vi "TestCHampSonde(2C).vi"(0 "Range":dbl=52.8 format="%.2f", 1 "CentreTel X":i32=647041 min=0 max=1000000 step=1000, 3 "PulsexCentre":i32=641444 min=0 max=1000000 step=1000, 5 "ParametresInstrumentaux":string[](array[string]), 9 "Rot(rad)":dbl=3.6441621315637374 step=0.1 format="%.2f", 11 "acrmin/pulse":dbl=5.28e-05 format="%.4e", 12 "CentreTel Y":i32=70736 min=0 max=1000000 step=1000, 14 "PulseyCentre":i32=41801 min=0 max=1000000 step=1000) -> (4 "Champ":cluster{dbl[], dbl[]}[](array[cluster])=[{[5.0, 5.0], [5.0, -5.0]}, {[5.0, -5.0], [-5.0, -5.0]}, {[-5.0, -5.0], [-5.0, 5.0]}, {[-5.0, 5.0], [5.0, 5.0]}, {[40.96033829233336, 15.527693293631083], [-35.21795510048486, 11.053208364139456]}, {[15.527693293631083, -30.74347017099323], [11.053208364139456, -14.37943663456282]}, {[-30.74347017099323, -5.310825172290953], [-14.37943663456282, -60.65060009918713]}, {[40.96033829233336, -5.310825172290953], [-35.21795510048486, -60.65060009918713]}, {array[360 elements], array[360 elements]}] {"?" format="%.2f"; "?" format="%.2f"}, 6 "offRA":dbl=0.9948732849489528 format="%.2f", 8 "rayon de sécurité ...":dbl, 10 "offDEC":dbl=-1.196509600791168 format="%.2f")   [LabVIEW 2010]
panel:
  out "p2y":dbl
  out "p2x":dbl
  out "p1y":dbl
  out "p1x":dbl
  out "XY Graph":cluster{dbl[], dbl[]}[](graph)
  # "Exclusion y1"
  # "Exclusion y2"
  # "Champ"
  # "Exclusion x1"
  # "Exclusion x2"
  # "foyerTel"
  # "foyerSonde"
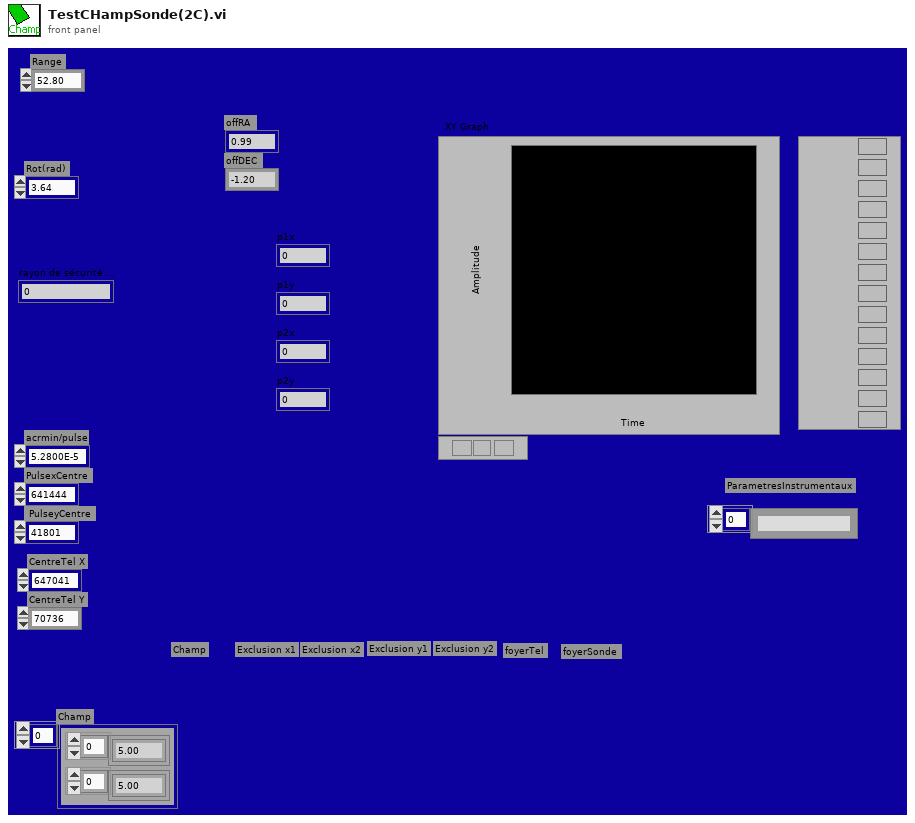
[diagram p1: front panel]
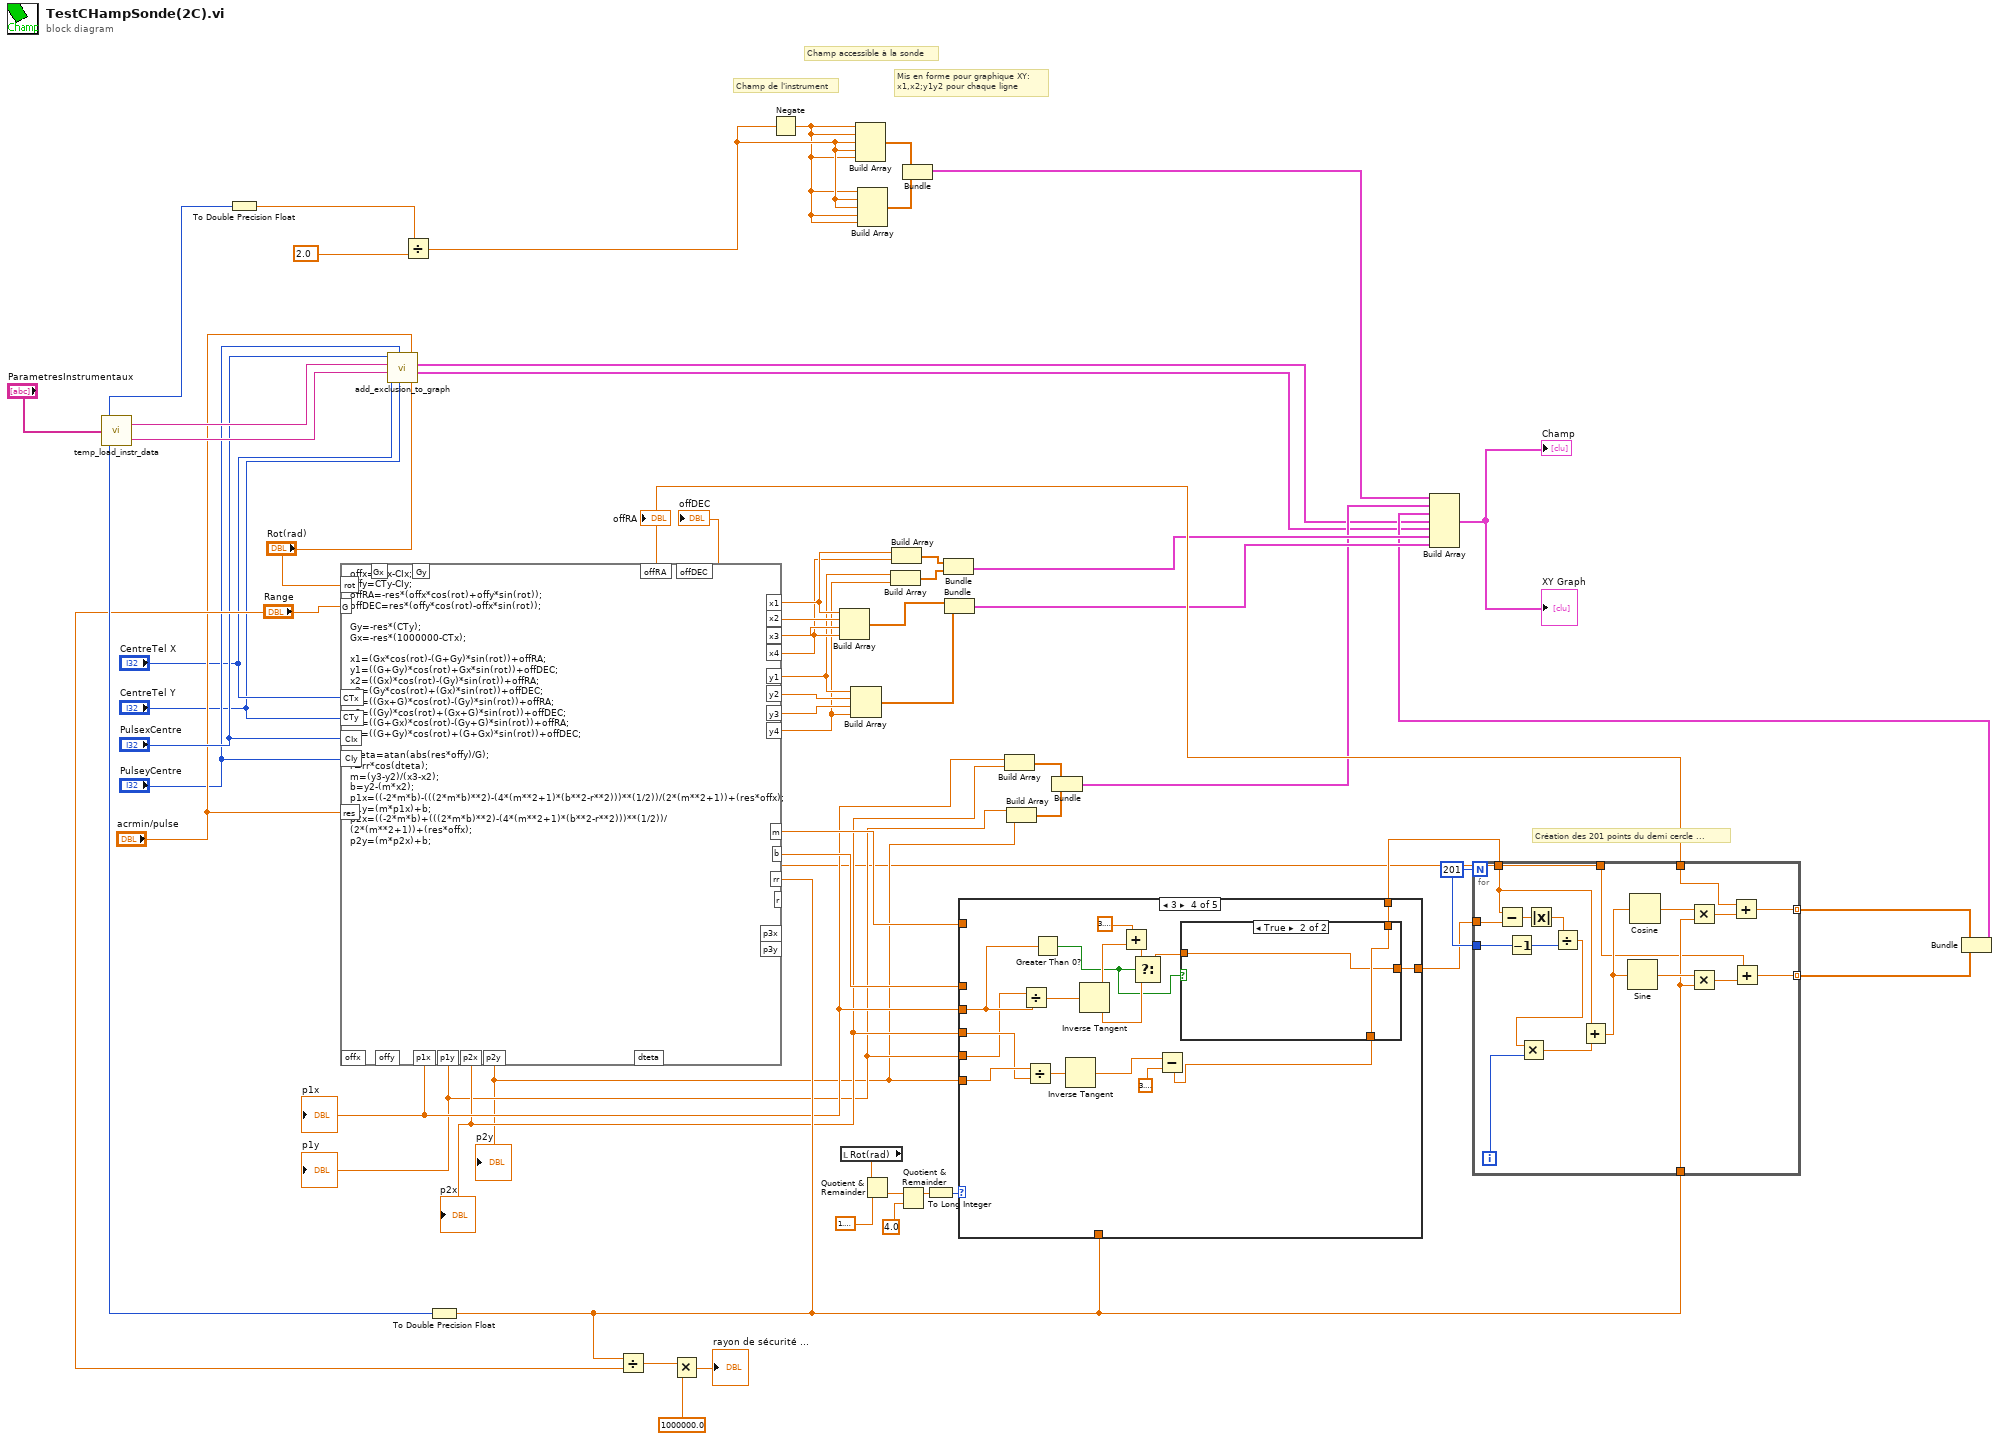
[diagram p0: block diagram]
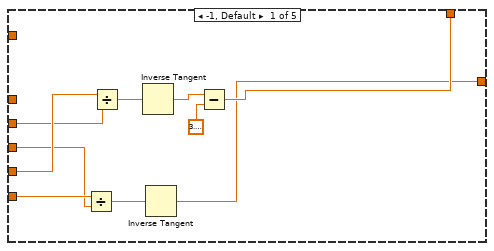
[diagram p2: hidden frame]
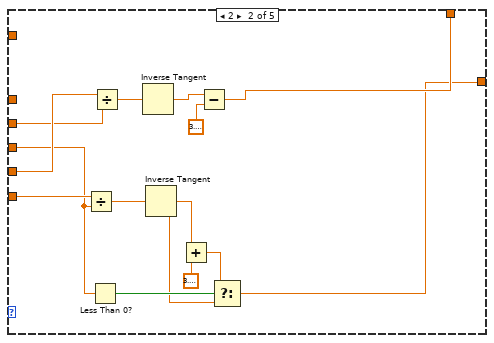
[diagram p3: hidden frame]
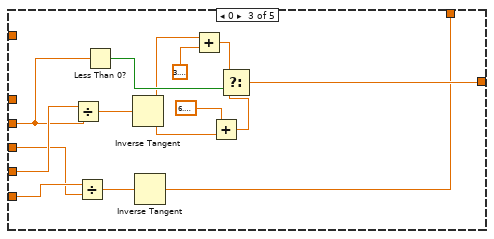
[diagram p4: hidden frame]
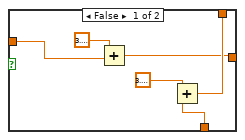
[diagram p5: hidden frame]
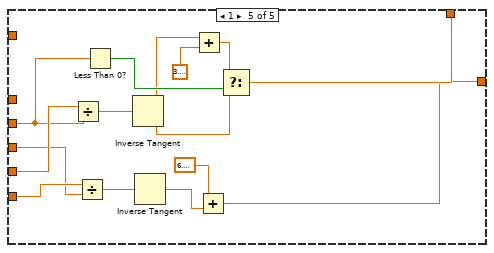
[diagram p6: hidden frame]
diagram:
  w59 = 201
  # "Création des 201 points du demi cercle ..."
  # "Champ accessible à la sonde"
  # "Champ de l'instrument"
  # "Mis en forme pour graphique XY:\nx1,x2;y1y2 pour chaque ligne"
  n1 = call "temp_load_instr_data.vi"("ParametresInstrumentaux"="ParametresInstrumentaux") -> ("2e couple"=w10:string, "1er couple"=w9:string, "rayon"=w46:i32, "champ"=w48:i32)
  n2 = To Double Precision Float(number=w48) -> (double precision float=w47:dbl)
  n3 = call "add_exclusion_to_graph.vi"("Rot(rad)"="Rot(rad)", "acrmin/pulse"="acrmin/pulse", "CentreTel Y"="CentreTel Y", "PulseyCentre"="PulseyCentre", "CentreTel X"="CentreTel X", "2er couple"=w10, "1er couple"=w9, "PulsexCentre"="PulsexCentre") -> ("Cavenas"=w1:cluster{dbl[], dbl[]}, "line one"=w2:cluster{dbl[], dbl[]})
  n4 = Divide(x=w47, y=2.0) -> (x/y=w36:dbl)
  n5 = To Double Precision Float(number=w46) -> (double precision float=w45:dbl)
  n6 = formula code="offx=CTx-CIx;\noffy=CTy-CIy;\noffRA=-res*(offx*cos(rot)+offy*sin(rot));\noffDEC=res*(offy*cos(rot)-offx*sin(rot));\n\nGy=-res*(CTy);\nGx=-res*(1000000-CTx);\n\nx1=(Gx*cos(rot)-(G+Gy)*sin(rot))+offRA;\ny1=((G+Gy)*cos(rot)+Gx*sin(rot))+offDEC;\nx2=((Gx)*cos(rot)-(Gy)*sin(rot))+offRA;\ny2=(Gy*cos(rot)+(Gx)*sin(rot))+offDEC;\nx3=((Gx+G)*cos(rot)-(Gy)*sin(rot))+offRA;\ny3=((Gy)*cos(rot)+(Gx+G)*sin(rot))+offDEC;\nx4=((G+Gx)*cos(rot)-(Gy+G)*sin(rot))+offRA;\ny4=((G+Gy)*cos(rot)+(G+Gx)*sin(rot))+offDEC;\n\ndteta=atan(abs(res*offy)/G);\nr=rr*cos(dteta);\nm=(y3-y2)/(x3-x2);\nb=y2-(m*x2);\np1x=((-2*m*b)-(((2*m*b)**2)-(4*(m**2+1)*(b**2-r**2)))**(1/2))/(2*(m**2+1))+(res*offx);\np1y=(m*p1x)+b;\np2x=((-2*m*b)+(((2*m*b)**2)-(4*(m**2+1)*(b**2-r**2)))**(1/2))/(2*(m**2+1))+(res*offx);\np2y=(m*p2x)+b;"("rot"="Rot(rad)", "CTx"="CentreTel X", "CTy"="CentreTel Y", "CIx"="PulsexCentre", "CIy"="PulseyCentre", "res"="acrmin/pulse", "G"="Range", "rr"=w45) -> ("x1"=w26:dbl, "x2"=w32:dbl, "y1"=w22:dbl, "y2"=w30:dbl, "x3"=w31:dbl, "x4"=w23:dbl, "y3"=w29:dbl, "y4"=w21:dbl, "offRA"=w20:dbl, "offDEC"=w19:dbl, "m"=w55:dbl, "b"=w56:dbl, "p1x"=w40:dbl, "p1y"=w38:dbl, "p2x"=w39:dbl, "p2y"=w37:dbl)  [unwired: 8 out]
  "offRA" <- w20
  "offDEC" <- w19
  "p1x" <- w40
  "p1y" <- w38
  "p2x" <- w39
  "p2y" <- w37
  n7 = Divide(x=w45, y="Range") -> (x/y=w44:dbl)
  n8 = Multiply(x=w44, y=1000000.0) -> (x*y=→"rayon de sécurité ...":dbl)
  n9 = Negate(x=w36) -> (-x=w35:dbl)
  n10 = Build Array(w26, w32, w31, w23) -> (w28:dbl[])
  n11 = local read "Rot(rad)"() -> (w54:dbl)
  n12 = Build Array(w22, w30, w29, w21) -> (w27:dbl[])
  n13 = Build Array(w35, w35, w36, w36, w35) -> (w33:dbl[])
  n14 = Build Array(w35, w36, w36, w35, w35) -> (w34:dbl[])
  n15 = Quotient & Remainder(x=w54, y=1.5707963267948966) -> (floor(x/y)=w51:dbl)  [unwired: 1 out]
  n16 = Build Array(w22, w21) -> (w24:dbl[])
  n17 = Build Array(w26, w23) -> (w25:dbl[])
  n18 = Quotient & Remainder(x=w51, y=4.0) -> (x-y*floor(x/y)=w49:dbl)  [unwired: 1 out]
  n19 = Bundle(w33, w34) -> (w12:cluster{dbl[], dbl[]})  [unwired: 1 in]
  n20 = To Long Integer(number=w49) -> (32bit integer=w52:i32)
  n21 = Bundle(w25, w24) -> (w18:cluster{dbl[], dbl[]})  [unwired: 1 in]
  n22 = Bundle(w28, w27) -> (w17:cluster{dbl[], dbl[]})  [unwired: 1 in]
  n23 = case shown="3" w52 {
    tunnel: w56 -> [_ _ _ _ _]
    tunnel: w55 -> [_ _ _ _ _]
    tunnel: [w73 w87 w88 w107 w129] -> w58
    tunnel: [w72 w74 w93 w106 w126] -> w57
    tunnel: w37 -> [w71 w86 w99 w117 w137]
    tunnel: w38 -> [w70 w85 w100 w104 w138]
    tunnel: w39 -> [w69 w79 w98 w116 w136]
    tunnel: w40 -> [w68 w84 w95 w105 w133]
    tunnel: w45 -> [_ _ _ _ _]
    frame -1, Default {
      n24 = Divide(x=w71, y=w69) -> (x/y=w64:dbl)
      n25 = Divide(x=w70, y=w68) -> (x/y=w67:dbl)
      n26 = Inverse Tangent(1:w67) -> (0:w66:dbl)
      n27 = Inverse Tangent(1:w64) -> (0:w72:dbl)
      n28 = Subtract(x=w66, y=3.141592653589793) -> (x-y=w73:dbl)
    }
    frame 2 {
      n29 = Divide(x=w86, y=w79) -> (x/y=w80:dbl)
      n30 = Less Than 0?(x=w79) -> (x < 0?=w78:bool)
      n31 = Divide(x=w85, y=w84) -> (x/y=w83:dbl)
      n32 = Inverse Tangent(1:w83) -> (0:w82:dbl)
      n33 = Inverse Tangent(1:w80) -> (0:w76:dbl)
      n34 = Add(x=w76, y=3.141592653589793) -> (x+y=w75:dbl)
      n35 = Subtract(x=w82, y=3.141592653589793) -> (x-y=w87:dbl)
      n36 = Select(t=w75, s=w78, f=w76) -> (s? t:f=w74:dbl)
    }
    frame 0 {
      n37 = Divide(x=w100, y=w95) -> (x/y=w101:dbl)
      n38 = Divide(x=w99, y=w98) -> (x/y=w97:dbl)
      n39 = Less Than 0?(x=w95) -> (x < 0?=w92:bool)
      n40 = Inverse Tangent(1:w101) -> (0:w89:dbl)
      n41 = Inverse Tangent(1:w97) -> (0:w88:dbl)
      n42 = Add(x=w89, y=3.141592653589793) -> (x+y=w94:dbl)
      n43 = Add(x=6.283185307179586, y=w89) -> (x+y=w90:dbl)
      n44 = Select(t=w94, s=w92, f=w90) -> (s? t:f=w93:dbl)
    }
    frame 3 {
      n45 = Divide(x=w104, y=w105) -> (x/y=w115:dbl)
      n46 = Divide(x=w117, y=w116) -> (x/y=w114:dbl)
      n47 = Greater Than 0?(x=w105) -> (x > 0?=w109:bool)
      n48 = Inverse Tangent(1:w114) -> (0:w103:dbl)
      n49 = Inverse Tangent(1:w115) -> (0:w112:dbl)
      n50 = Add(x=3.141592653589793, y=w112) -> (x+y=w111:dbl)
      n51 = Select(t=w111, s=w109, f=w112) -> (s? t:f=w108:dbl)
      n52 = Subtract(x=w103, y=3.141592653589793) -> (x-y=w102:dbl)
      n53 = case shown="True" w109 {
        tunnel: w102 -> [w121 w125]
        tunnel: w108 -> [w119 w124]
        tunnel: [w120 w125] -> w107
        tunnel: [w118 w124] -> w106
        frame False {
          n54 = Add(x=3.141592653589793, y=w119) -> (x+y=w118:dbl)
          n55 = Add(x=3.141592653589793, y=w121) -> (x+y=w120:dbl)
        }
        frame True {
        }
      }
    }
    frame 1 {
      n56 = Divide(x=w138, y=w133) -> (x/y=w139:dbl)
      n57 = Divide(x=w137, y=w136) -> (x/y=w135:dbl)
      n58 = Less Than 0?(x=w133) -> (x < 0?=w131:bool)
      n59 = Inverse Tangent(1:w139) -> (0:w130:dbl)
      n60 = Inverse Tangent(1:w135) -> (0:w127:dbl)
      n61 = Add(x=w130, y=3.141592653589793) -> (x+y=w132:dbl)
      n62 = Add(x=6.283185307179586, y=w127) -> (x+y=w126:dbl)
      n63 = Select(t=w132, s=w131, f=w130) -> (s? t:f=w129:dbl)
    }
  }
  n64 = Build Array(w40, w39) -> (w61:dbl[])
  n65 = Build Array(w38, w37) -> (w60:dbl[])
  n66 = Bundle(w61, w60) -> (w13:cluster{dbl[], dbl[]})  [unwired: 1 in]
  n67 = for {
    N: w59 -> [_]
    tunnel: [w145] -> w16 mode=indexing
    tunnel: [w142] -> w15 mode=indexing
    tunnel: w45 -> [w156]
    tunnel: w58 -> [w150]
    tunnel: w57 -> [w155]
    tunnel: w59 -> [w154]
    tunnel: w20 -> [w144]
    tunnel: w19 -> [w141]
    i -> [w153]
    n68 = Subtract(x=w150, y=w155) -> (x-y=w148:dbl)
    n69 = Decrement(x=w154) -> (x-1=w140:i32)
    n70 = Absolute Value(x=w148) -> (abs(x)=w147:dbl)
    n71 = Divide(x=w147, y=w140) -> (x/y=w152:dbl)
    n72 = Multiply(x=w152, y=w153) -> (x*y=w151:dbl)
    n73 = Add(x=w150, y=w151) -> (x+y=w149:dbl)
    n74 = Sine(x=w149) -> (sin(x)=w157:dbl)
    n75 = Cosine(x=w149) -> (cos(x)=w158:dbl)
    n76 = Multiply(x=w158, y=w156) -> (x*y=w146:dbl)
    n77 = Multiply(x=w157, y=w156) -> (x*y=w143:dbl)
    n78 = Add(x=w144, y=w146) -> (x+y=w145:dbl)
    n79 = Add(x=w141, y=w143) -> (x+y=w142:dbl)
  }
  n80 = Bundle(w16, w15) -> (w14:cluster{dbl[], dbl[]})  [unwired: 1 in]
  n81 = Build Array(w12, w13, w14, w2, w1, w18, w17) -> (→"Champ" →"XY Graph":cluster{dbl[], dbl[]}[])
